vi "Read Config.vi"(8 "error in (no error)":errorcluster, 10 "Resource In":variant, 11 "Analyze Parameter Fluence in":refnum<class "Analyze Parameter Fluence.lvclass">) -> (0 "error out":errorcluster, 2 "Resource Out":variant, 3 "Analyze Parameter Fluence out":refnum<class "Analyze Parameter Fluence.lvclass">)   [LabVIEW 2020, in "Analyze Parameter Fluence.lvclass"]
uses:
  Analyze Parameter Fluence.lvclass
  C:/POLARIS Programme/POLARIS-AS-3-Cams/Submodules/HIJ Vision/Analyze/Analyze Parameter/Analyze Parameter Base/Analyze Parameter Base.lvclass
  <vilib>/Utility/config.llb/Config Data RefNum.ctl
  Analyze Parameter Fluence.lvclass/Analyze Parameter Fluence.ctl
  <vilib>/Utility/config.llb/Read Key (I32).vi
  <vilib>/Utility/config.llb/NI_LVConfig.lvlib
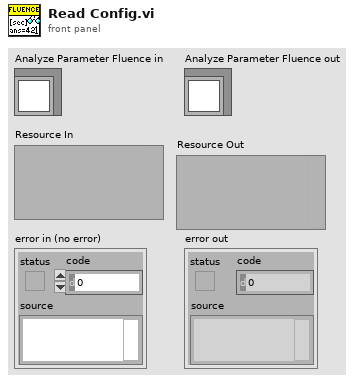
[diagram p1: front panel]
types:
  T1 = typedef "NI_LVConfig.lvlib/Config Data RefNum.ctl" = refnum<k1>
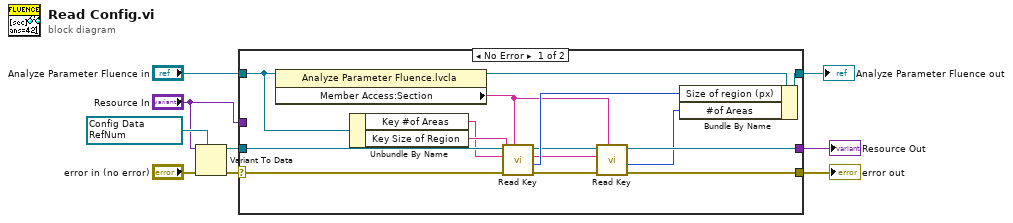
[diagram p0: block diagram]
diagram:
  w9 = T1 refnum items=["config data"] ("refnum")
  n1 = Variant To Data(error in="error in (no error)", type=w9, Variant="Resource In") -> (data=w8:T1, error out=w7:errorcluster)
  n2 = case shown="No Error" w7 {
    selector: w7 -> [w17 w25]
    tunnel: w8 -> [w23 _]
    tunnel: "Analyze Parameter Fluence in" -> [w18 w24]
    tunnel: [w21 w24] -> w3
    tunnel: [w13 w26] -> w2
    tunnel: [w11 w25] -> w1
    tunnel: "Resource In" -> [_ w26]
    frame No Error {
      n3 = property class="Analyze Parameter Fluence.lvcla"(reference=w18) -> (reference out=w19:refnum<class "Analyze Parameter Fluence.lvclass">, "Member Access:Section"=w15:string)  [unwired: 1 in, 1 out]
      n4 = Unbundle By Name(w18) -> ("Key #of Areas"=w16:string, "Key Size of Region"=w20:string)
      n5 = call-poly <vilib>:"Read Key.vi"("section"=w15, "error in (no error)"=w17, "key"=w20, "refnum"=w23) -> ("error out"=w12:errorcluster, "value"=w22:i32, "refnum out"=w14:T1)  [unwired: 4 in, 1 out]
      n6 = call-poly <vilib>:"Read Key.vi"("section"=w15, "error in (no error)"=w12, "key"=w16, "refnum"=w14) -> ("error out"=w11:errorcluster, "value"=w10:i32, "refnum out"=w13:T1)  [unwired: 4 in, 1 out]
      n7 = Bundle By Name(cluster=w19, "Size of region (px)"=w22, "#of Areas"=w10) -> (w21:refnum<class "Analyze Parameter Fluence.lvclass">)
    }
    frame Error {
    }
  }
  "error out" <- w1
  "Analyze Parameter Fluence out" <- w3
  "Resource Out" <- w2
